vi "123.vi"(0 "机械臂末端姿态":dbl[][](array[numeric]), 1 "逆运动学输入":dbl[](array[numeric])=[0.2, 0.0, 0.3]) -> (2 "1231":dbl[](array[numeric]), 3 "1232":dbl[](array[numeric]), 4 "1233":dbl[](array[numeric]), 5 "1234":dbl[](array[numeric]))   [LabVIEW 2015]
uses:
  <vilib>/Utility/file.llb/Read From Spreadsheet File (DBL).vi
panel:
  out "angle12":dbl
  out "抓手长度":dbl
  out "123b":dbl[](array[numeric])
  out "123a":dbl[](array[numeric])
  out "angle24":dbl
  out "angle23":dbl
  out "angle32":dbl
  out "angle31":dbl
  out "angle22":dbl
  out "angle21":dbl
  out "角度/弧度":dbl
  out "弧度/角度":dbl
  out "az":dbl=1.0
  out "ay":dbl
  out "ax":dbl
  out "angle3":dbl
  out "angle2":dbl
  out "angle1":dbl
  out "逆运动学输出":dbl[](array[numeric])=[0.0, 90.0, 0.0, 0.0, -90.0, -0.0] format="%#.3f"
  in  "机械臂臂长":dbl[](array[numeric])=[558.0, 764.0, 993.0, 420.0]
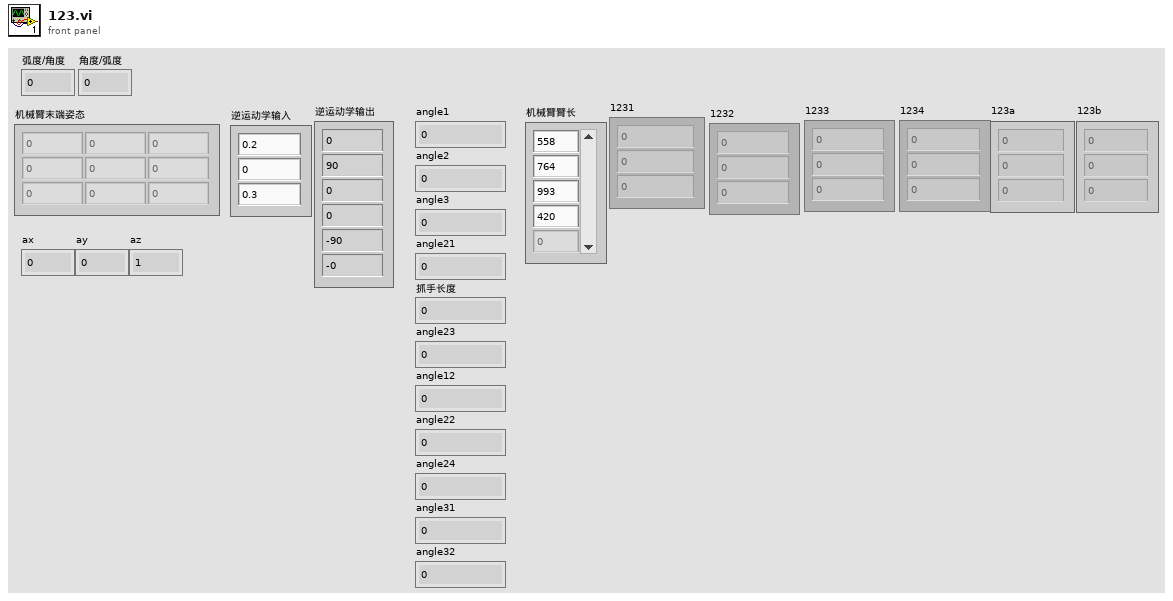
[diagram p1: front panel]
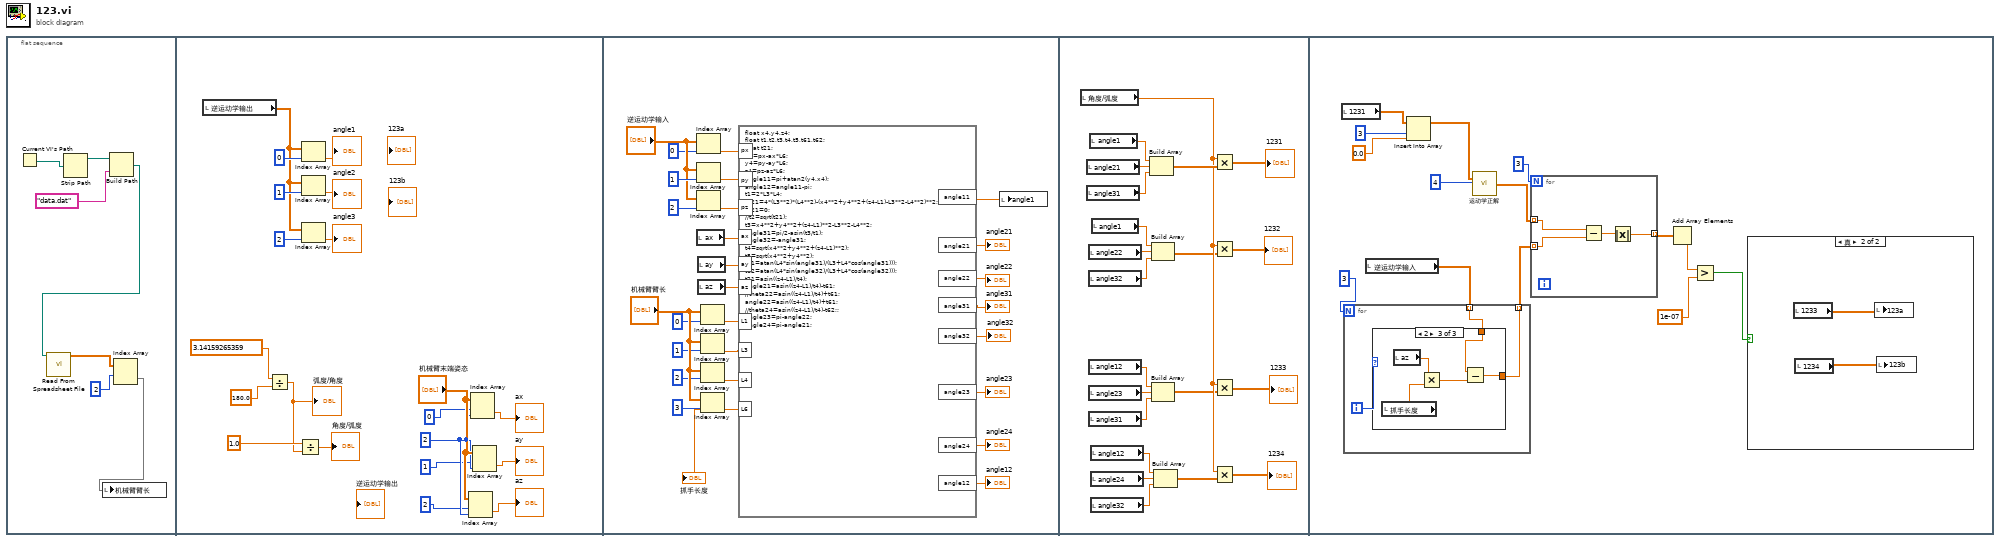
[diagram p0: block diagram]
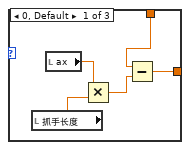
[diagram p2: hidden frame]
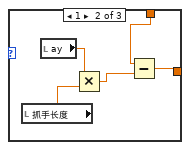
[diagram p3: hidden frame]
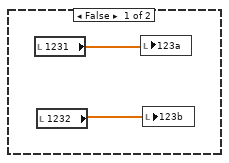
[diagram p4: hidden frame]
diagram:
  n1 = flat-sequence {
    frame #0 {
      n2 = Current VI's Path() -> (path=w4:path)
      n3 = Strip Path(path=w4) -> (stripped path=w3:path)  [unwired: 1 out]
      n4 = Build Path(base path=w3, name or relative path="data.dat") -> (appended path=w1:path)
      n5 = call-poly <vilib>:"Read From Spreadsheet File.vi"("file path (dialog if empty)"=w1) -> ("all rows"=w7:dbl[][])  [unwired: 6 in, 4 out]
      n6 = Index Array(array=w7, index (row)=2) -> (element=w6:dbl[])  [unwired: 1 in]
      n7 = local write "机械臂臂长"(w6) -> ()
    }
    frame #1 {
      w17 = 2
      n8 = local read "逆运动学输出"() -> (w21:dbl[])
      n9 = Divide(x=3.14159265359, y=180.0) -> (x/y=w9:dbl)
      "弧度/角度" <- w9
      n10 = Divide(x=1.0, y=w9) -> (x/y=→"角度/弧度":dbl)
      n11 = Index Array(array=w21, index=0) -> (element=→"angle1":dbl)
      n12 = Index Array(array=w21, index=1) -> (element=→"angle2":dbl)
      n13 = Index Array(array=w21, index=2) -> (element=→"angle3":dbl)
      n14 = Index Array(array="机械臂末端姿态", index (row)=2, index (col)=w17) -> (element=→"az":dbl)
      n15 = Index Array(array="机械臂末端姿态", index (row)=0, index (col)=w17) -> (element=→"ax":dbl)
      n16 = Index Array(array="机械臂末端姿态", index (row)=1, index (col)=w17) -> (element=→"ay":dbl)
    }
    frame #2 {
      n17 = Index Array(array="逆运动学输入", index=0) -> (element=w40:dbl)
      n18 = Index Array(array="逆运动学输入", index=1) -> (element=w41:dbl)
      n19 = Index Array(array="逆运动学输入", index=2) -> (element=w42:dbl)
      n20 = local read "ax"() -> (w51:dbl)
      n21 = local read "ay"() -> (w52:dbl)
      n22 = local read "az"() -> (w53:dbl)
      n23 = Index Array(array="机械臂臂长", index=0) -> (element=w47:dbl)
      n24 = Index Array(array="机械臂臂长", index=1) -> (element=w48:dbl)
      n25 = Index Array(array="机械臂臂长", index=2) -> (element=w49:dbl)
      n26 = Index Array(array="机械臂臂长", index=3) -> (element=w50:dbl)
      "抓手长度" <- w50
      n27 = formula code="float x4,y4,z4;\nfloat t1,t2,t3,t4,t5,t61,t62;\nfloat t21;\nx4=px-ax*L6;\ny4=py-ay*L6;\nz4=pz-az*L6;\nangle11=pi+atan2(y4,x4);\nangle12=angle11-pi;\nt1=2*L3*L4;\n//t21=4*(L3**2)*(L4**2)-(x4**2+y4**2+(z4-L1)-L3**2-L4**2)**2;\n//t21=0;\n//t2=sqrt(t21);\nt3=x4**2+y4**2+(z4-L1)**2-L3**2-L4**2;\nangle31=pi/2-asin(t3/t1);\nangle32=-angle31;\nt4=sqrt(x4**2+y4**2+(z4-L1)**2);\nt5=sqrt(x4**2+y4**2);\nt61=atan(L4*sin(angle31)/(L3+L4*cos(angle31)));\nt62=atan(L4*sin(angle32)/(L3+L4*cos(angle32)));\nt21=asin((z4-L1)/t4);\nangle21=asin((z4-L1)/t4)-t61;\n//theta22=asin((z4-L1)/t4)+t61;\nangle22=asin((z4-L1)/t4)+t61;\n//theta24=asin((z4-L1)/t4)-t62;;\nangle23=pi-angle22;\nangle24=pi-angle21;"("px"=w40, "py"=w41, "pz"=w42, "L1"=w47, "L3"=w48, "L4"=w49, "L6"=w50, "ax"=w51, "ay"=w52, "az"=w53) -> ("angle11"=w35:dbl, "angle21"=→"angle21":dbl, "angle32"=→"angle32":dbl, "angle31"=→"angle31":dbl, "angle22"=→"angle22":dbl, "angle23"=→"angle23":dbl, "angle24"=→"angle24":dbl, "angle12"=→"angle12":dbl)
      n28 = local write "angle1"(w35) -> ()
    }
    frame #3 {
      n29 = local read "角度/弧度"() -> (w61:dbl)
      n30 = local read "angle21"() -> (w74:dbl)
      n31 = local read "angle31"() -> (w73:dbl)
      n32 = local read "angle22"() -> (w71:dbl)
      n33 = local read "angle32"() -> (w72:dbl)
      n34 = local read "angle12"() -> (w69:dbl)
      n35 = local read "angle23"() -> (w68:dbl)
      n36 = local read "angle31"() -> (w67:dbl)
      n37 = local read "angle1"() -> (w75:dbl)
      n38 = local read "angle12"() -> (w64:dbl)
      n39 = local read "angle24"() -> (w65:dbl)
      n40 = local read "angle32"() -> (w66:dbl)
      n41 = local read "angle1"() -> (w70:dbl)
      n42 = Build Array(w75, w74, w73) -> (w63:dbl[])
      n43 = Build Array(w70, w71, w72) -> (w60:dbl[])
      n44 = Build Array(w69, w68, w67) -> (w59:dbl[])
      n45 = Build Array(w64, w65, w66) -> (w58:dbl[])
      n46 = Multiply(x=w61, y=w63) -> (x*y=→"1231":dbl[])
      n47 = Multiply(x=w61, y=w60) -> (x*y=→"1232":dbl[])
      n48 = Multiply(x=w61, y=w59) -> (x*y=→"1233":dbl[])
      n49 = Multiply(x=w61, y=w58) -> (x*y=→"1234":dbl[])
    }
    frame #4 {
      n50 = local read "1231"() -> (w89:dbl[])
      n51 = local read "逆运动学输入"() -> (w77:dbl[])
      n52 = for {
        N: 3 -> [_]
        tunnel: w77 -> [w92] mode=indexing
        tunnel: [w90] -> w76 mode=indexing
        i -> [w91]
        n53 = case shown="2" w91 {
          tunnel: w92 -> [w93 w98 w103]
          tunnel: [w94 w99 w105] -> w90
          frame 0, Default {
            n54 = local read "抓手长度"() -> (w96:dbl)
            n55 = local read "ax"() -> (w97:dbl)
            n56 = Multiply(x=w97, y=w96) -> (x*y=w95:dbl)
            n57 = Subtract(x=w93, y=w95) -> (x-y=w94:dbl)
          }
          frame 1 {
            n58 = local read "抓手长度"() -> (w102:dbl)
            n59 = local read "ay"() -> (w101:dbl)
            n60 = Multiply(x=w101, y=w102) -> (x*y=w100:dbl)
            n61 = Subtract(x=w98, y=w100) -> (x-y=w99:dbl)
          }
          frame 2 {
            n62 = local read "抓手长度"() -> (w106:dbl)
            n63 = local read "az"() -> (w107:dbl)
            n64 = Multiply(x=w107, y=w106) -> (x*y=w104:dbl)
            n65 = Subtract(x=w103, y=w104) -> (x-y=w105:dbl)
          }
        }
      }
      n66 = Insert Into Array(array=w89, index=3, new element=0.0) -> (w86:dbl[])
      n67 = call "运动学正解.vi"("正运动学输入"=w86, "关节数"=4) -> ("正解输出"=w83:dbl[])  [unwired: 2 out]
      n68 = for {
        N: 3 -> [_]
        tunnel: w83 -> [w115] mode=indexing
        tunnel: w76 -> [w114] mode=indexing
        tunnel: [w112] -> w82 mode=indexing
        n69 = Subtract(x=w115, y=w114) -> (x-y=w113:dbl)
        n70 = Absolute Value(x=w113) -> (abs(x)=w112:dbl)
      }
      n71 = Add Array Elements(numeric array=w82) -> (sum=w81:dbl)
      n72 = Greater?(x=w81, y=1e-07) -> (0:w79:bool)
      n73 = case shown="真" w79 {
        frame False {
          n74 = local read "1231"() -> (w109:dbl[])
          n75 = local read "1232"() -> (w108:dbl[])
          n76 = local write "123a"(w109) -> ()
          n77 = local write "123b"(w108) -> ()
        }
        frame True {
          n78 = local read "1233"() -> (w111:dbl[])
          n79 = local read "1234"() -> (w110:dbl[])
          n80 = local write "123a"(w111) -> ()
          n81 = local write "123b"(w110) -> ()
        }
      }
    }
  }
